vi "Create Sysdef Tree from DB Channel Clusters_RTs.vi"(7 "Autocreate Rx timestamp chans?":bool, 8 "error in":errorcluster, 10 "RTs":T1[](array[typedef]), 11 "Device Ptr":u64) -> (0 "error out":errorcluster)   [LabVIEW 2017, in "Ballard 1553 System Explorer.lvlib"]
uses:
  Ballard 1553 System Explorer.lvlib
  Parse XML Ballard/Ballard_RT.ctl
  Parse XML Ballard/Ballard_RT subAddress.ctl
  Parse XML Ballard/Ballard_RT direction.ctl
  Parse XML Ballard/Ballard_RT rtMode.ctl
  Parse XML Ballard/Ballard_RT modeCode.ctl
  <vilib>/NI Veristand/Custom Device API/Custom Device Channel.ctl
  <vilib>/NI Veristand/Custom Device API/Custom Device Channel Type.ctl
  Shared/Controls and Global/Global.vi
  <vilib>/NI Veristand/Custom Device API/Set Item Property (I32).vi
  <vilib>/NI Veristand/Custom Device API/Set Item Property (U16).vi
  <vilib>/NI VeriStand/Custom Device API/Custom Device API.lvlib
  Shared/Ballard 1553 Shared.lvlib
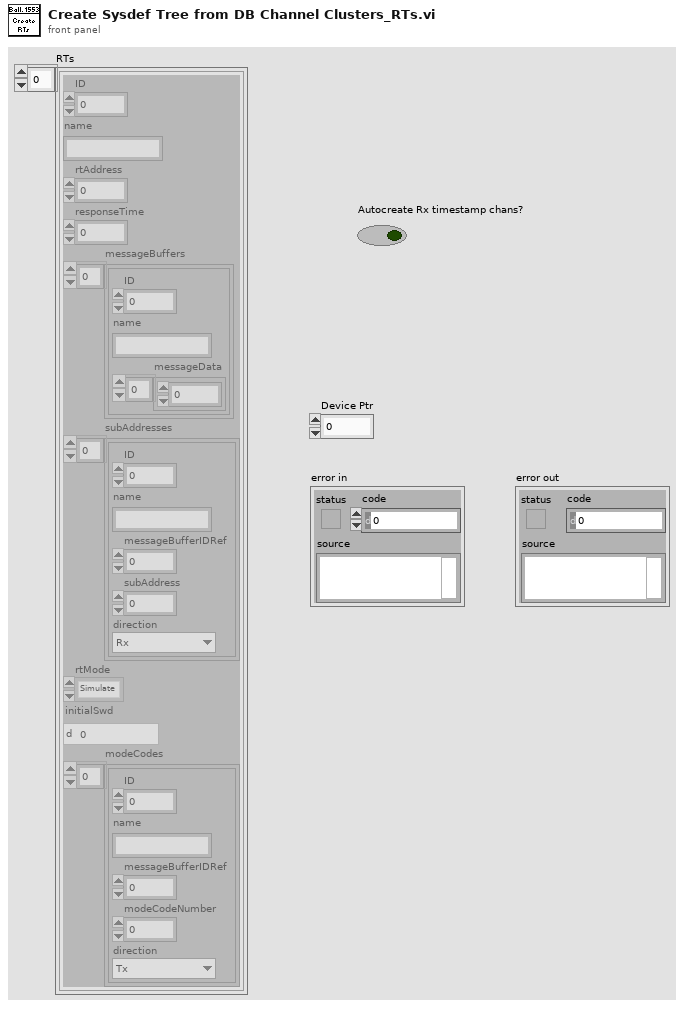
[diagram p1: front panel]
types:
  T1 = typedef "Ballard 1553 System Explorer.lvlib/Ballard_RT.ctl" = cluster{"ID":i32, "name":string, "rtAddress":i8, "responseTime":i32, "messageBuffers":cluster{"ID":i32, "name":string, "messageData":u16[]}[], "subAddresses":T2[], "rtMode":T4, "initialSwd":u16, "modeCodes":T5[]}
  T2 = typedef "Ballard 1553 System Explorer.lvlib/Ballard_RT subAddress.ctl" = cluster{"ID":i32, "name":string, "messageBufferIDRef":i32, "subAddress":i8, "direction":T3}
  T3 = typedef "Ballard 1553 System Explorer.lvlib/Ballard_RT direction.ctl" = enum16{"Tx", "Rx"}
  T4 = typedef "Ballard 1553 System Explorer.lvlib/Ballard_RT rtMode.ctl" = enum16{"Simulate", "Monitor", "Disable"}
  T5 = typedef "Ballard 1553 System Explorer.lvlib/Ballard_RT modeCode.ctl" = cluster{"ID":i32, "name":string, "messageBufferIDRef":i32, "modeCodeNumber":i8, "direction":T3}
  T6 = enum16{"DW", "STC", "SPC", "SW", "TI MC", "AC", "TI WC"}
  T7 = typedef "Custom Device API.lvlib/Custom Device Channel Type.ctl" = enum16{"Input", "Output"}
  T8 = typedef "Custom Device API.lvlib/Custom Device Channel.ctl" = cluster{"Type":T7, "Units":string, "Default Value":dbl, "Faultable":bool, "Scalable":bool}
  T9 = cluster{"ID":i32, "name":string, "messageData":u16[]}[]
  T10 = typedef "Custom Device API.lvlib/Custom Device Item Ref.ctl" = u64
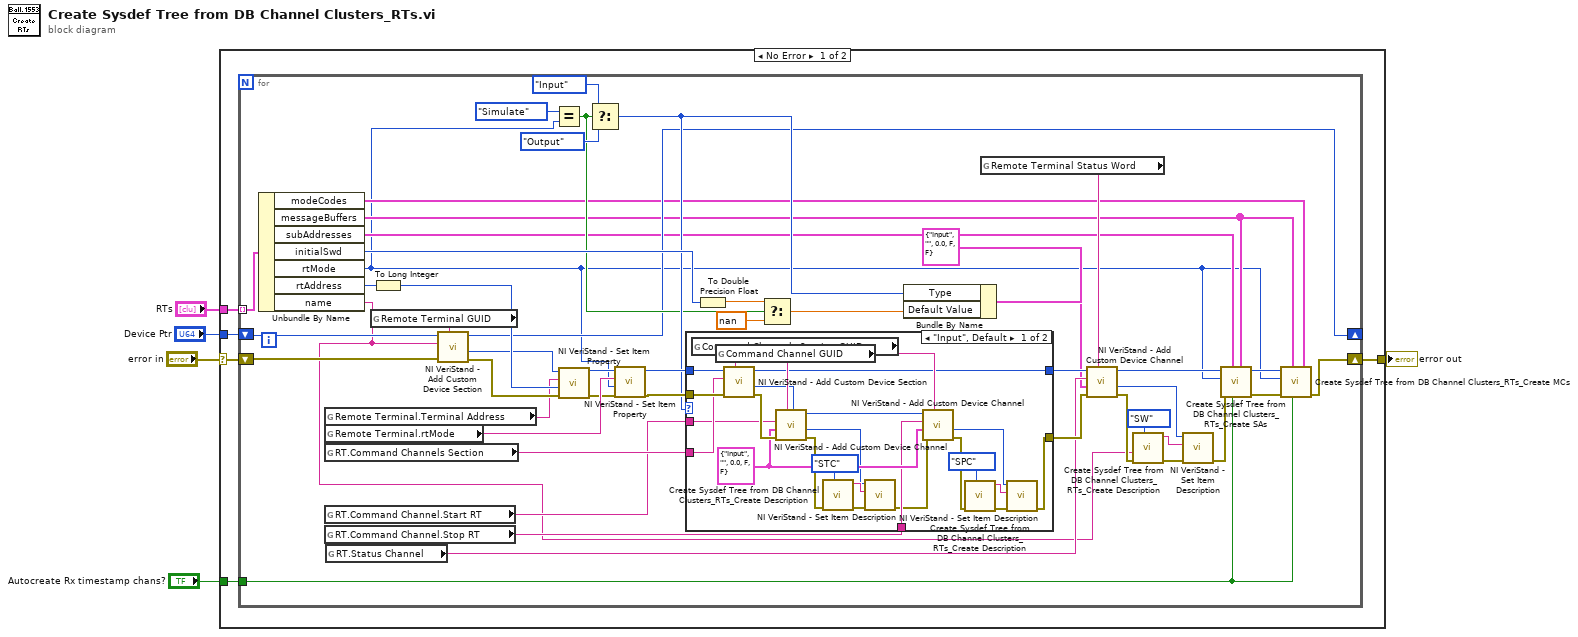
[diagram p0: block diagram]
diagram:
  n1 = case shown="No Error" "error in" {
    selector: "error in" -> [w9 w85]
    tunnel: [w8 w85] -> w4
    tunnel: "Device Ptr" -> [w10 _]
    tunnel: "RTs" -> [w6 _]
    tunnel: "Autocreate Rx timestamp chans?" -> [w7 _]
    frame No Error {
      n2 = for {
        tunnel: w6 -> [w58] mode=indexing
        shift-right: [w23] -> w8
        shift-left: w9 -> [w29]
        tunnel: w7 -> [w18]
        shift-right: [w30] -> _
        shift-left: w10 -> [w28]
        n3 = Unbundle By Name(w58) -> ("modeCodes"=w21:T5[], "messageBuffers"=w22:T9, "subAddresses"=w24:T2[], "initialSwd"=w40:u16, "rtMode"=w20:T4, "rtAddress"=w55:i8, "name"=w12:string)
        n4 = global read "Global.vi" "Remote Terminal.Terminal Address"() -> (w53:string)
        n5 = global read "Global.vi" "Remote Terminal.rtMode"() -> (w51:string)
        n6 = global read "Global.vi" "RT.Command Channels Section"() -> (w48:string)
        n7 = global read "Global.vi" "RT.Command Channel.Start RT"() -> (w47:string)
        n8 = global read "Global.vi" "RT.Command Channel.Stop RT"() -> (w46:string)
        n9 = global read "Global.vi" "RT.Status Channel"() -> (w43:string)
        n10 = global read "Global.vi" "Remote Terminal GUID"() -> (w57:string)
        n11 = To Long Integer(number=w55) -> (32bit integer=w54:i32)
        n12 = call <vilib>:"NI VeriStand - Add Custom Device Section.vi"("GUID (Default Section)"=w57, "error in (no error)"=w29, "Section Name"=w12, "Parent Ref in"=w28) -> ("error out"=w56:errorcluster, "Section Ptr"=w19:T10, "Parent Ref out"=w30:T10)  [unwired: 4 in, 1 out]
        n13 = Equal?(x=Ballard_RT_rtMode."Simulate", y=w20) -> (x = y?=w32:bool)
        n14 = call-poly <vilib>:"NI VeriStand - Set Item Property.vi"("error in (no error)"=w56, "Value"=w54, "Property Name"=w53, "Item Ref in"=w19) -> ("error out"=w49:errorcluster, "Item Ref out"=w52:T10)  [unwired: 5 in, 1 out]
        n15 = Select(t=Custom_Device_Channel_Type."Input" ("Type"), s=w32, f=Custom_Device_Channel_Type."Output") -> (s? t:f=w35:T7)
        n16 = call-poly <vilib>:"NI VeriStand - Set Item Property.vi"("Value"=w20, "Property Name"=w51, "Item Ref in"=w52) -> ("Item Ref out"=w50:T10)  [unwired: 6 in, 2 out]
        n17 = case shown="\"Input\", Default" w35 {
          tunnel: w50 -> [w77 w84]
          tunnel: w49 -> [w76 w83]
          tunnel: w48 -> [w75 _]
          tunnel: w47 -> [w74 _]
          tunnel: w46 -> [w73 _]
          tunnel: [w72 w84] -> w45
          tunnel: [w64 w83] -> w44
          frame "Input", Default {
            w78 = T8 {"Type"=enum."Input", "Units"="", "Default Value"=0.0, "Faultable"=FALSE, "Scalable"=FALSE} ("Channel")
            n18 = global read "Global.vi" "Command Channels Section GUID"() -> (w71:string)
            n19 = global read "Global.vi" "Command Channel GUID"() -> (w82:string)
            n20 = call <vilib>:"NI VeriStand - Add Custom Device Section.vi"("GUID (Default Section)"=w71, "error in (no error)"=w76, "Section Name"=w75, "Parent Ref in"=w77) -> ("error out"=w80:errorcluster, "Section Ptr"=w79:T10, "Parent Ref out"=w72:T10)  [unwired: 4 in, 1 out]
            n21 = call <vilib>:"NI VeriStand - Add Custom Device Channel.vi"("GUID (Default Channel)"=w82, "error in (no error)"=w80, "Channel"=w78, "Channel Name"=w74, "Parent Ref in"=w79) -> ("error out"=w70:errorcluster, "Channel Ref"=w62:T10, "Parent Ref out"=w81:T10)  [unwired: 3 in, 1 out]
            n22 = call "Create Sysdef Tree from DB Channel Clusters_RTs_Create Description.vi"("Type"=T6."STC", "error in (no error)"=w70) -> ("error out"=w69:errorcluster, "Description (Out)"=w68:string)  [unwired: 8 in]
            n23 = call <vilib>:"NI VeriStand - Set Item Description.vi"("error in (no error)"=w69, "Description"=w68, "Item Ref in"=w62) -> ("error out"=w63:errorcluster)  [unwired: 6 in, 2 out]
            n24 = call <vilib>:"NI VeriStand - Add Custom Device Channel.vi"("GUID (Default Channel)"=w82, "error in (no error)"=w63, "Channel"=w78, "Channel Name"=w73, "Parent Ref in"=w81) -> ("error out"=w65:errorcluster, "Channel Ref"=w61:T10)  [unwired: 3 in, 2 out]
            n25 = call "Create Sysdef Tree from DB Channel Clusters_RTs_Create Description.vi"("Type"=T6."SPC", "error in (no error)"=w65) -> ("error out"=w66:errorcluster, "Description (Out)"=w67:string)  [unwired: 8 in]
            n26 = call <vilib>:"NI VeriStand - Set Item Description.vi"("error in (no error)"=w66, "Description"=w67, "Item Ref in"=w61) -> ("error out"=w64:errorcluster)  [unwired: 6 in, 2 out]
          }
          frame "Output" {
          }
        }
        n27 = To Double Precision Float(number=w40) -> (double precision float=w33:dbl)
        n28 = Select(t=w33, s=w32, f=nan) -> (s? t:f=w34:dbl)
        n29 = Bundle By Name(cluster=T8 {"Type"=enum."Input", "Units"="", "Default Value"=0.0, "Faultable"=FALSE, "Scalable"=FALSE} ("Channel"), "Type"=w35, "Default Value"=w34) -> (w41:T8)
        n30 = global read "Global.vi" "Remote Terminal Status Word"() -> (w39:string)
        n31 = call <vilib>:"NI VeriStand - Add Custom Device Channel.vi"("GUID (Default Channel)"=w39, "error in (no error)"=w44, "Channel"=w41, "Channel Name"=w43, "Parent Ref in"=w45) -> ("error out"=w16:errorcluster, "Channel Ref"=w13:T10, "Parent Ref out"=w25:T10)  [unwired: 3 in, 1 out]
        n32 = call "Create Sysdef Tree from DB Channel Clusters_RTs_Create Description.vi"("Type"=T6."SW", "error in (no error)"=w16, "Name"=w12) -> ("error out"=w17:errorcluster, "Description (Out)"=w15:string)  [unwired: 7 in]
        n33 = call <vilib>:"NI VeriStand - Set Item Description.vi"("error in (no error)"=w17, "Description"=w15, "Item Ref in"=w13) -> ("error out"=w14:errorcluster)  [unwired: 6 in, 2 out]
        n34 = call "Create Sysdef Tree from DB Channel Clusters_RTs_Create SAs.vi"("messageBuffers"=w22, "Autocreate Rx timestamp chans?"=w18, "subAddresses"=w24, "error in (no error)"=w14, "rtMode"=w20, "Section Ptr in"=w25) -> ("error out"=w27:errorcluster, "Section Ptr out"=w26:T10)  [unwired: 4 in]
        n35 = call "Create Sysdef Tree from DB Channel Clusters_RTs_Create MCs.vi"("modeCodes"=w21, "Autocreate Rx timestamp chans?"=w18, "messageBuffers"=w22, "error in (no error)"=w27, "rtMode"=w20, "Section Ptr in"=w26) -> ("error out"=w23:errorcluster)  [unwired: 5 in]
      }
    }
    frame Error {
    }
  }
  "error out" <- w4
